vi "SLSC Create Property Path String.vi"(9 "Datatype":string, 10 "Property":string, 11 "Physical Channel":string) -> (3 "SLSC Path String":string)   [LabVIEW 2015, in "SLSC CD Shared.lvlib"]
uses:
  SLSC CD Shared.lvlib
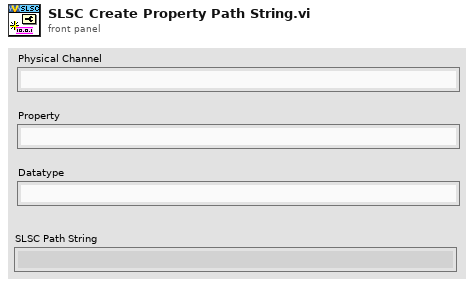
[diagram p1: front panel]
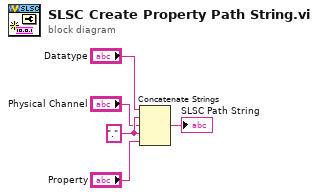
[diagram p0: block diagram]
diagram:
  w4 = "." ("string")
  n1 = Concatenate Strings("Datatype", w4, "Physical Channel", w4, "Property") -> (→"SLSC Path String":string)
